vi "Test Run Suite of Suites.vi"(8 "error in (no error)":errorcluster, 11 "Test Case In":refnum<class "LUnit Test Suite Tests.lvclass">) -> (0 "error out":errorcluster, 3 "Test Case Out":refnum<class "LUnit Test Suite Tests.lvclass">)   [LabVIEW 2020, in "LUnit Test Suite Tests.lvclass"]
uses:
  LUnit Test Suite Tests.lvclass
  C:/Program Files (x86)/National Instruments/LabVIEW 2020/vi.lib/Astemes/LUnit/Test Case.lvclass
  Test Case Test Double/Test Case Test Double.lvclass
  C:/Git/astemes-lunit/source/API/LUnit Test Case/LUnit Test Case.lvclass
  <vilib>/Astemes/LUnit/Test Case.lvclass/Test Case.ctl
  b74e4934-f044-4222-b3dd-fc90e6c1bd4f.vi
  <vilib>/Astemes/LUnit/Palette/Pass.vi
  <vilib>/Astemes/LUnit/Palette/Fail.vi
  <vilib>/Astemes/LUnit/Compare Variants.vi
  <vilib>/Astemes/LUnit/Describe Comparison.vi
  <vilib>/Astemes/LUnit/Set Assertion Type.vi
  <vilib>/Astemes/LUnit/Add test result.vi
  <vilib>/Astemes/LUnit/Variant to string.vi
  <vilib>/Astemes/LUnit/LUnit Record Assertion Result.vi
  <vilib>/Astemes/LUnit/LUnit Aggregate Assertion Results.vi
  <vilib>/Astemes/LUnit/Method Result/LUnit Merge Status.vi
  <vilib>/Astemes/LUnit/LUnit Concatenate result strings.vi
  source/API/LUnit Test Suite/LUnit Test Suite.lvclass
  C:/Git/astemes-lunit/source/Core/Runnable/Runnable.lvclass
  <vilib>/Utility/Data Type/Get Type Information.vi
  <vilib>/Utility/LVClass/Get LV Class Name.vi
  source/Core/Runnable/Runnable.lvclass
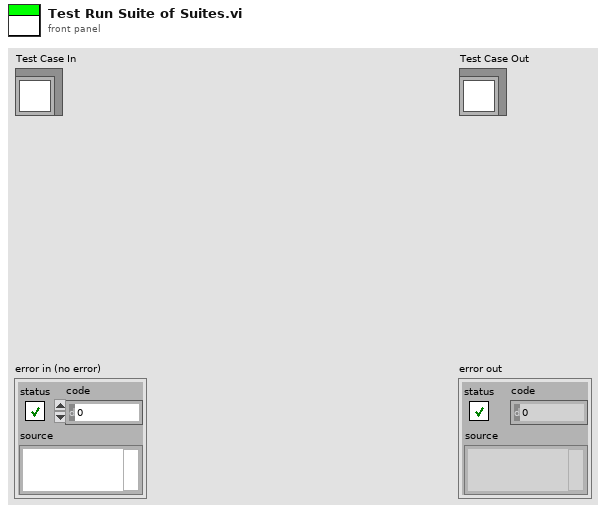
[diagram p1: front panel]
types:
  T1 = typedef "Result.lvlib/Result.ctl" = cluster{"Name":string, "Message":string, "Description":string, "Status":T2, "Result Type":T3, "Execution Time":dbl}
  T2 = typedef "Result.lvlib/Status.ctl" = enum16{"", "Passed", "Failed", "Error", "Skipped", "Setup Error", "Broken", "Teardown Error"}
  T3 = typedef "Result.lvlib/Type.ctl" = enum16{"Method", "Case", "Suite", "Pass", "Fail", "Skip", "Pass if", "Fail if", "Pass if Error", "Fail if Error", "Pass if Equal", "Fail if Equal"}
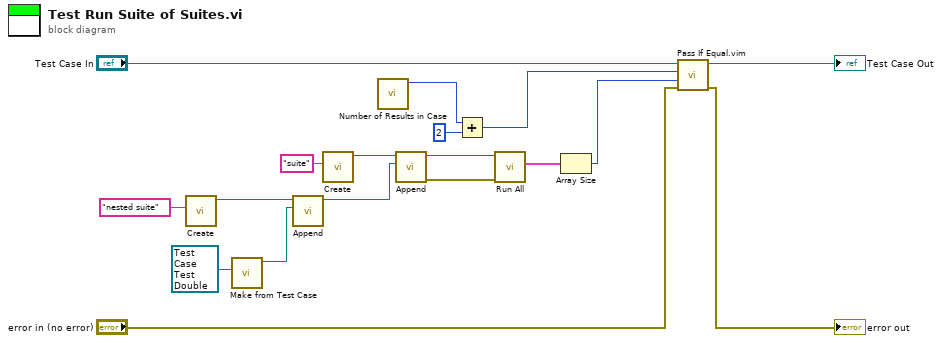
[diagram p0: block diagram]
diagram:
  n1 = call "Create.vi"("Suite Name"="nested suite" ("Name")) -> ("LUnit Test Suite Out"=w4:refnum<class "LUnit Test Suite.lvclass">)  [unwired: 9 in, 1 out]
  n2 = call "Make from Test Case.vi"("LUnit Test Case"=refnum<class "Test Case Test Double.lvclass"> refnum ("LUnit Test Case V2 Test Double.lvclass")) -> ("LUnit Test Suite Out"=w3:refnum<class "LUnit Test Suite.lvclass">)  [unwired: 9 in, 1 out]
  n3 = call "Append.vi"("Runnable"=w3, "LUnit Test Suite In"=w4) -> ("LUnit Test Suite Out"=w6:refnum<class "LUnit Test Suite.lvclass">)  [unwired: 8 in, 1 out]
  n4 = call "Create.vi"("Suite Name"="suite") -> ("LUnit Test Suite Out"=w2:refnum<class "LUnit Test Suite.lvclass">)  [unwired: 9 in, 1 out]
  n5 = call "Number of Results in Case.vi"() -> ("Number of Results"=w8:i32)  [unwired: 11 in]
  n6 = call "Append.vi"("Runnable"=w6, "LUnit Test Suite In"=w2) -> ("error out"=w12:errorcluster, "LUnit Test Suite Out"=w11:refnum<class "LUnit Test Suite.lvclass">)  [unwired: 8 in]
  n7 = Add(x=w8, y=2 ("size(s)")) -> (x+y=w7:i32)
  n8 = call "Run All.vi"("error in (no error)"=w12, "Runnable In"=w11) -> ("Results"=w14:T1[])  [unwired: 8 in, 1 out]
  n9 = Array Size(array=w14) -> (size(s)=w13:i32)
  n10 = call "Pass If Equal.vim"("error in (no error)"="error in (no error)", "Actual"=w13, "Expected"=w7, "LUnit Test Case In"="Test Case In") -> ("error out"=→"error out":errorcluster, "LUnit Test Case Out"=→"Test Case Out":refnum<class "LUnit Test Suite Tests.lvclass">)  [unwired: 6 in]
